vi "Clear Waveform Chart History.vi"(8 "error in (no error)":errorcluster, 11 "references in":refnum<vi>) -> (0 "error out":errorcluster, 3 "references out":refnum<vi>)   [LabVIEW 2018]
doc: "Clears the history of referenced waveform charts. Currently only supports waveform charts with a 2D numeric double data type."
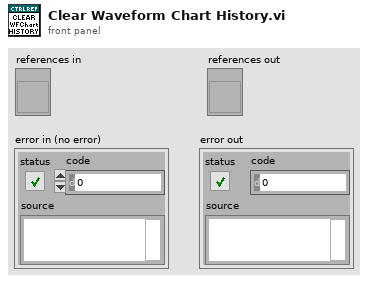
[diagram p1: front panel]
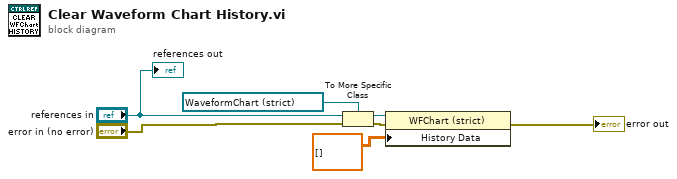
[diagram p0: block diagram]
diagram:
  n1 = To More Specific Class(target class=refnum<vi> refnum ("Waveform Chart"), reference="references in", error in="error in (no error)") -> (specific class reference=w3:refnum<vi>, error out=w2:errorcluster)
  n2 = property on="Property Node" class="WFChart (strict)"(reference=w3, error in=w2, "History Data"=dbl[][] []) -> (error out=→"error out":errorcluster)  [unwired: 1 out]
  "references out" <- "references in"
